vi "Practica5.vi"() -> ()   [LabVIEW 2017]
panel:
  out "Posición":cluster{"Y":dbl[], "Y":dbl[]}[](graph)
  in  "Agregar Datos":bool
  in  "x":dbl min=0.0 max=36.0 step=0.01
  in  "y":dbl min=0.0 max=70.0 step=0.01
  in  "Reset":bool
  # "Práctica 5: Ensayo de Templabilidad\n\nOBJETIVO: Determinar la templabilidad de un acero, mediante la\nprueba o ensayo de templabilidad o Ensayo JOMINY"
  # "LABORATORIO DE MATERIALES"
  # "LABORATORIO DE MATERIALES"
  # "OFF"
  # "ON"
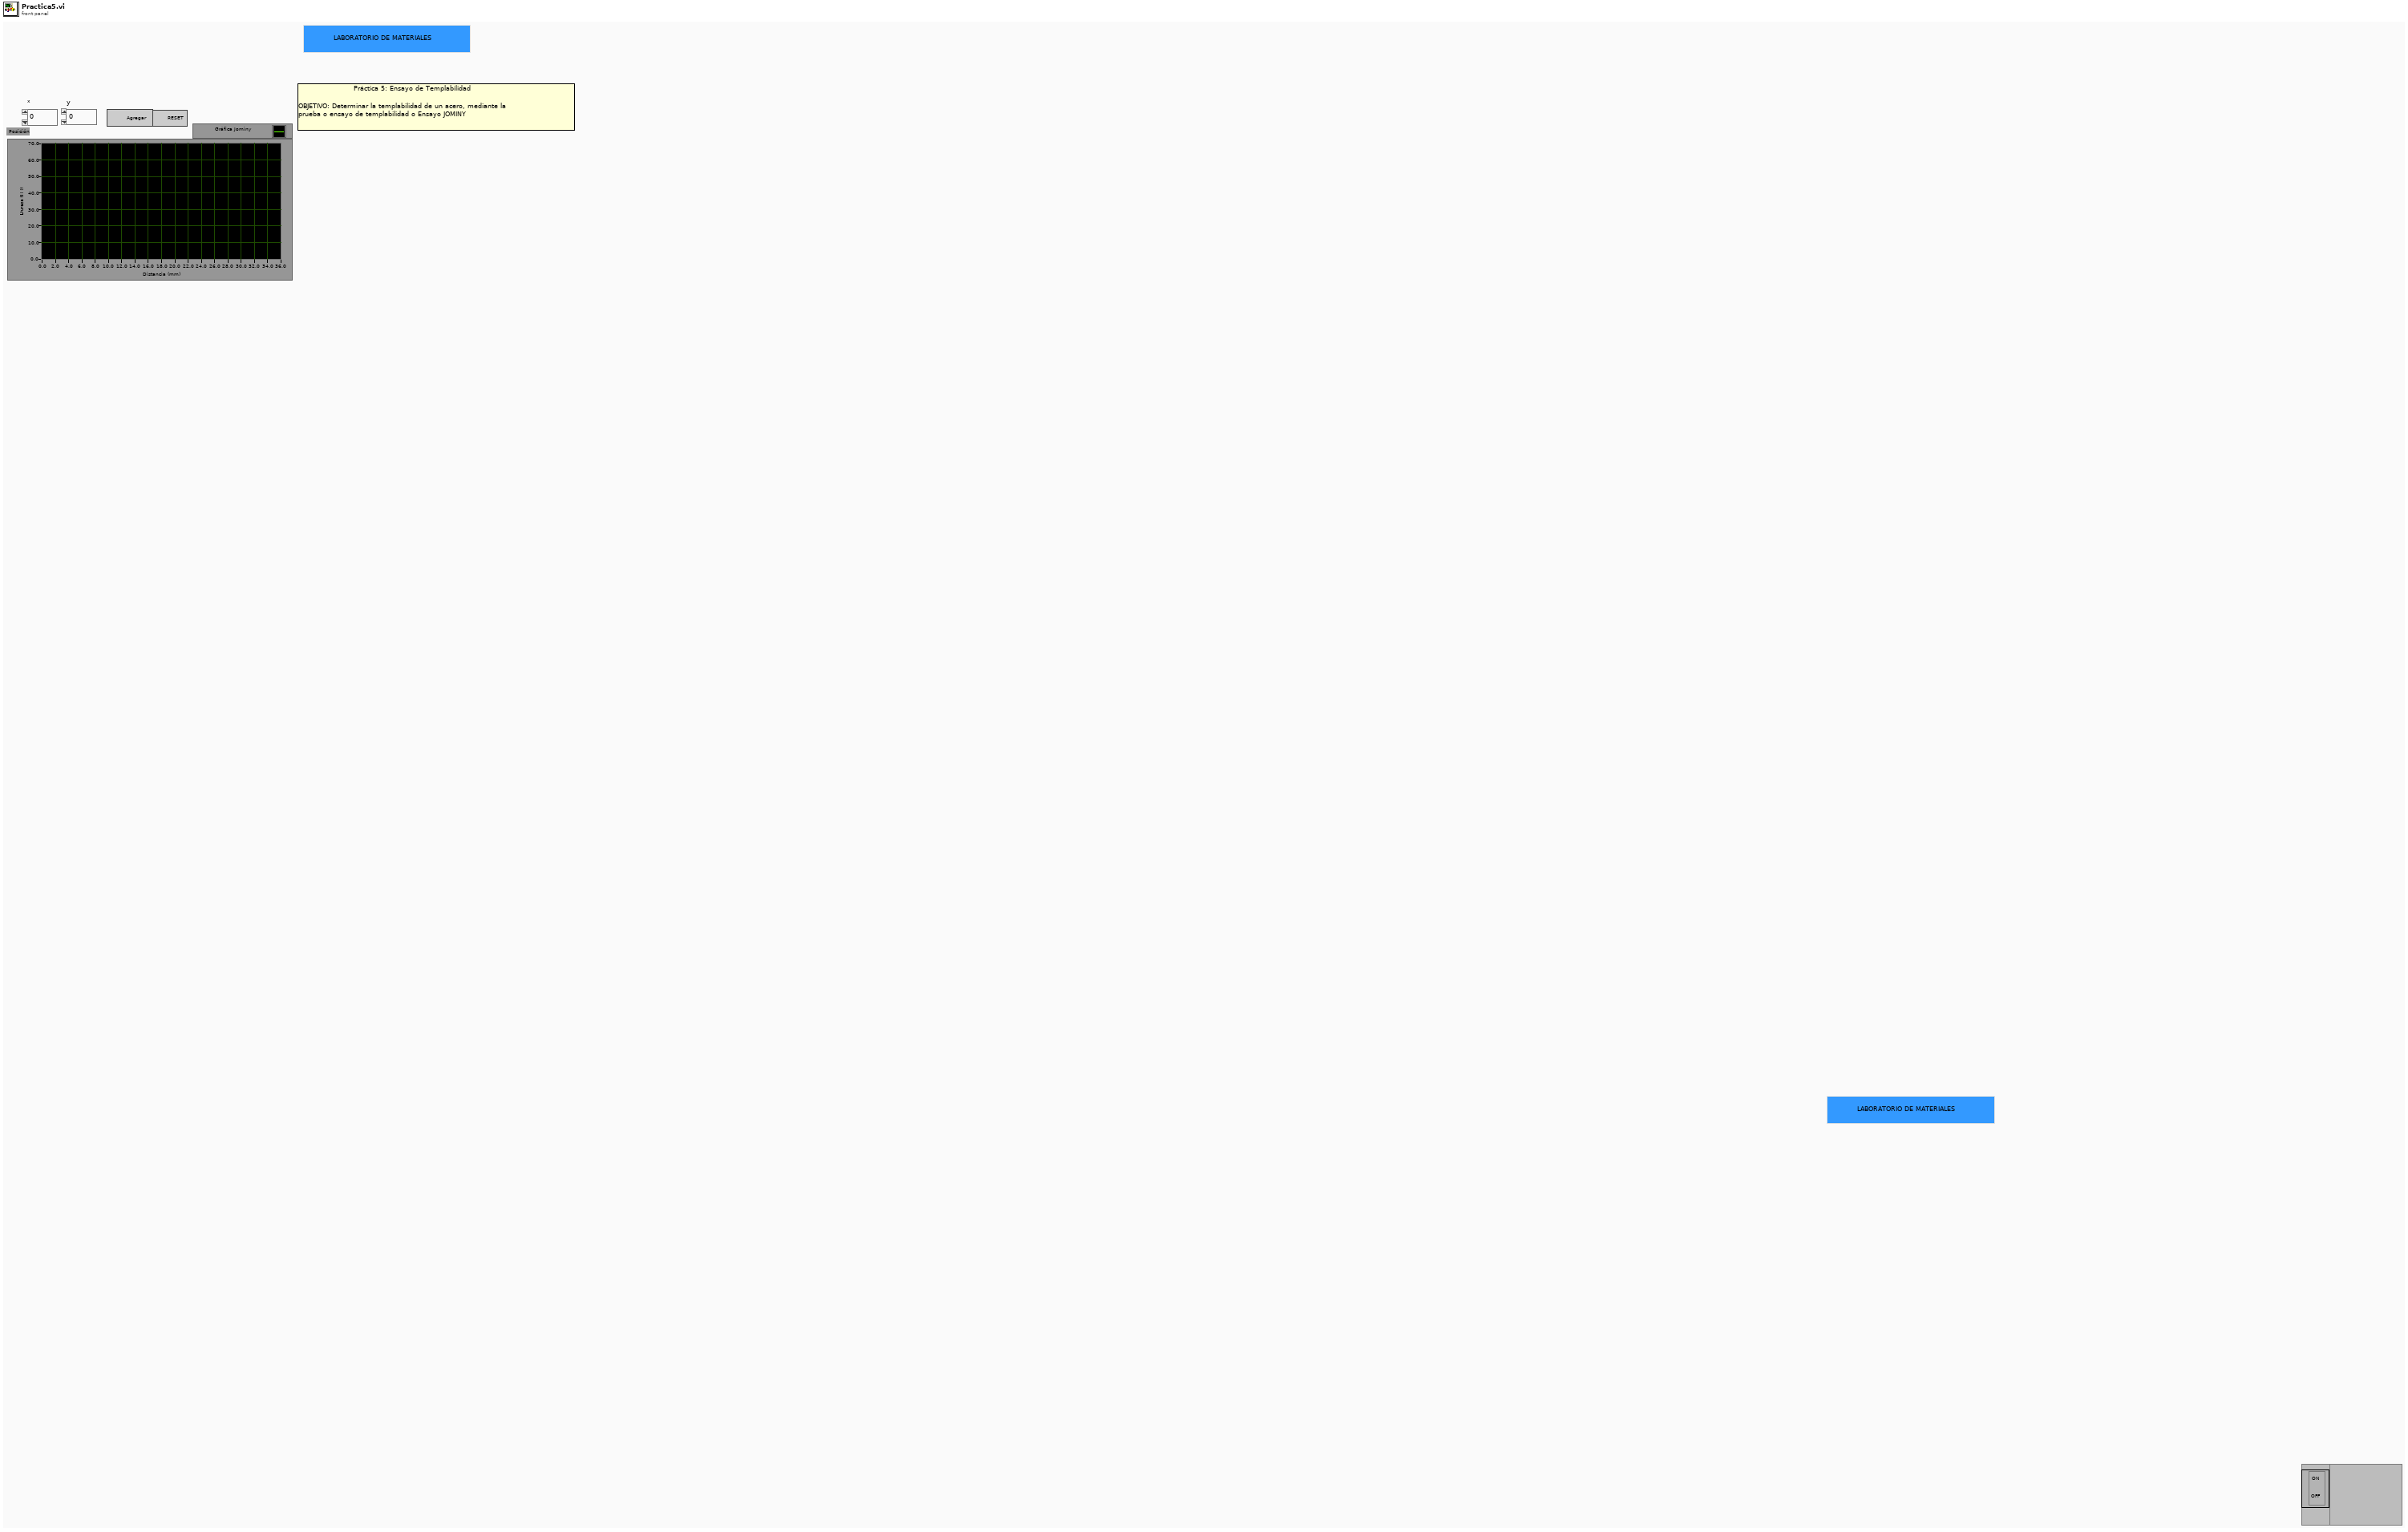
[diagram p1: front panel]
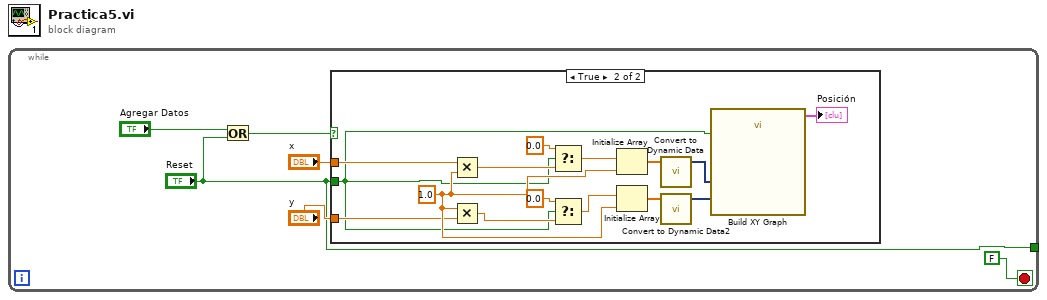
[diagram p0: block diagram]
diagram:
  n1 = while {
    tunnel: ["Reset"] -> _
    stop <- FALSE stop-if-true
    n2 = Or(x="Agregar Datos", y="Reset") -> (x .or. y?=w3:bool)
    n3 = case shown="True" w3 {
      tunnel: "x" -> [_ w15]
      tunnel: "y" -> [_ w14]
      tunnel: "Reset" -> [_ w7]
      frame False {
      }
      frame True {
        w16 = 1.0 ("y")
        n4 = Multiply(x=w15, y=w16) -> (x*y=w10:dbl)
        n5 = Multiply(x=w16, y=w14) -> (x*y=w11:dbl)
        n6 = Select(t=0.0, s=w7, f=w10) -> (s? t:f=w13:dbl)
        n7 = Select(t=0.0, s=w7, f=w11) -> (s? t:f=w12:dbl)
        n8 = Initialize Array(w13, w16) -> (w20:dbl[])
        n9 = Initialize Array(w12, w16) -> (w21:dbl[])
        n10 = call "Convert to Dynamic Data"("Array"=w20) -> ("Dynamic Data Type"=w17:dynamicdata)  [unwired: 3 in]
        n11 = call "Convert to Dynamic Data2"("Array"=w21) -> ("Dynamic Data Type"=w18:dynamicdata)  [unwired: 3 in]
        n12 = call "Build XY Graph"("Reset"=w7, "Y Input"=w18, "X Input"=w17) -> ("XY Graph"=→"Posición":cluster{"Y":dbl[], "Y":dbl[]}[])  [unwired: 2 in, 6 out]
      }
    }
  }
